vi "User Actor Core Close.vi"(0 "MainUI in":refnum<class "MainUI.lvclass">, 11 "Error in":errorcluster caption="Error in (no error)") -> (4 "MainUI out":refnum<class "MainUI.lvclass">, 15 "Error out":errorcluster)   [LabVIEW 2018, in "HOG MainUI.lvlib" / "MainUI.lvclass"]
doc: "Close custom resources opened during <B>Actor</B> initialization or run. Typical actions:\n\n- Close ActorCore window.\n\nKåre Juul Kirkegaard\nHOG Svømning\n3/4 2019"
uses:
  MainUI.lvclass
  MainUI.lvclass/MainUI.ctl
  <vilib>/GPower/UI/Library/GP UI.lvlib
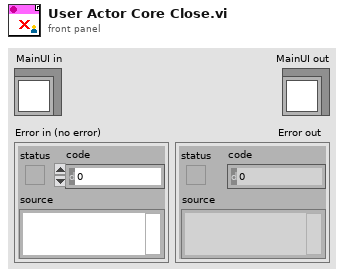
[diagram p1: front panel]
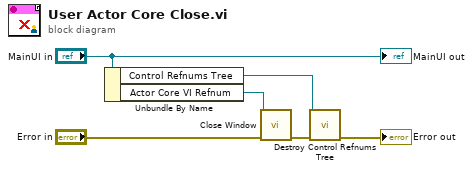
[diagram p0: block diagram]
diagram:
  n1 = Unbundle By Name("MainUI in") -> ("Control Refnums Tree"=w1:refnum<class "Dictionary.lvclass">, "Actor Core VI Refnum"=w4:refnum<vi>)
  n2 = call <vilib>:"Close Window.vi"("VI Refnum"=w4, "Error in"="Error in") -> ("Error out"=w3:errorcluster)  [unwired: 13 in]
  n3 = call <vilib>:"Destroy Control Refnums Tree.vi"("Control Refnums Tree"=w1, "Error in"=w3) -> ("Error out"=→"Error out":errorcluster)  [unwired: 13 in]
  "MainUI out" <- "MainUI in"
